vi "sv_Overall Level Plot (XY).vi"(6 "X axis selection":u16(ring)=2 items=["Time", "Revolution", "RPM"], 7 "reset? (True)":bool=TRUE, 8 "speed profile":T1 {"speed [RPM]" format="%.2f"; "time [s]" format="%.2f"}, 9 "samples/rev":dbl=1.0 format="%.2f", 11 "overall level (even angular)":dbl[][](array[numeric]) format="%.2f") -> (1 "X unit":string, 3 "overall level":cluster{"X":dbl[], "Y":dbl[]}[](array[cluster]) {"Y" format="%.2f"; "X" format="%.2f"})   [LabVIEW 2017, in "SoundVib_ContSweptSine.lvlib"]
uses:
  <vilib>/addons/Sound and Vibration/svt_Continuous Swept Sine/SoundVib_ContSweptSine.lvlib
  <vilib>/addons/Sound and Vibration/Order Analysis/Tach Process/SubVIs/speed profile.ctl
  <vilib>/Analysis/1siggen.llb/Ramp Pattern by Samples.vi
  <vilib>/Analysis/NI_AALBase.lvlib
  <vilib>/addons/Sound and Vibration/Order Analysis/Tach Process/SoundVib_TachProcess.lvlib
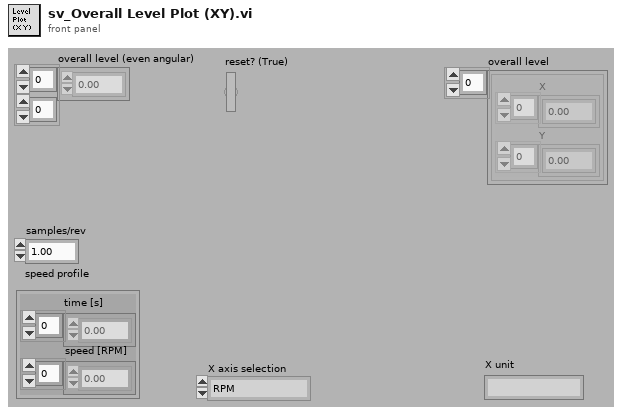
[diagram p1: front panel]
types:
  T1 = typedef "SoundVib_TachProcess.lvlib/speed profile.ctl" = cluster{"time [s]":dbl[], "speed [RPM]":dbl[]}
  T2 = cluster{"time [s]":dbl[], "overall level (even angular)":dbl[]}
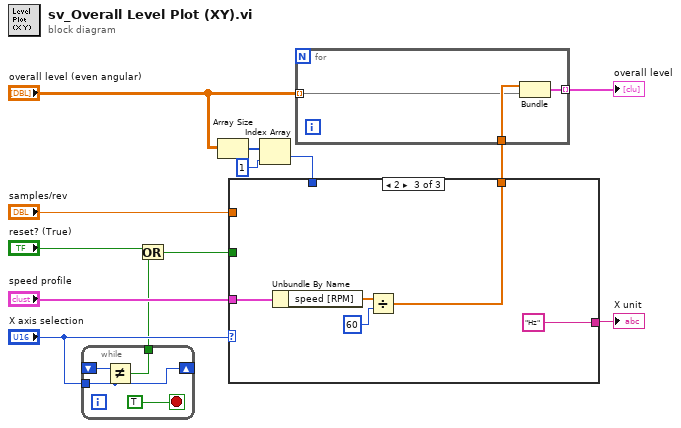
[diagram p0: block diagram]
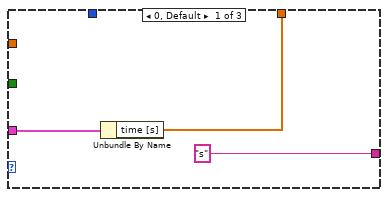
[diagram p2: hidden frame]
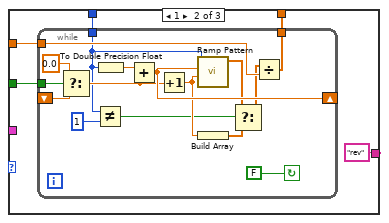
[diagram p3: hidden frame]
diagram:
  n1 = while {
    shift-right: [w15] -> _
    shift-left: _ -> [w16]
    tunnel: "X axis selection" -> [w15]
    tunnel: [w14] -> w1
    stop <- TRUE stop-if-true
    n2 = Not Equal?(x=w16, y=w15) -> (x != y?=w14:bool)
  }
  n3 = Or(x="reset? (True)", y=w1) -> (x .or. y?=w3:bool)
  n4 = Array Size(array="overall level (even angular)") -> (size(s)=w12:i32[])
  n5 = Index Array(array=w12, index=1) -> (element=w9:i32)
  n6 = case shown="2" "X axis selection" {
    tunnel: "speed profile" -> [w20 _ w46]
    tunnel: [w19 w25 w43] -> w10
    tunnel: w9 -> [_ w21 _]
    tunnel: "samples/rev" -> [_ w23 _]
    tunnel: ["s" "rev" "Hz"] -> w6
    tunnel: w3 -> [_ w22 _]
    frame 0, Default {
      n7 = Unbundle By Name(w20) -> ("time [s]"=w19:dbl[])
    }
    frame 1 {
      n8 = while {
        tunnel: [w41] -> w25
        tunnel: w23 -> [w40]
        tunnel: w22 -> [w38]
        shift-right: [w35] -> _
        shift-left: _ -> [w36]
        tunnel: w21 -> [w32]
        stop <- FALSE continue-if-true
        n9 = Select(t=0.0 ("f"), s=w38, f=w36) -> (s? t:f=w34:dbl)
        n10 = Not Equal?(x=w32, y=1) -> (x != y?=w30:bool)
        n11 = To Double Precision Float(number=w32) -> (double precision float=w26:dbl)
        n12 = Add(x=w26, y=w34) -> (x+y=w35:dbl)
        n13 = Increment(x=w34) -> (x+1=w31:dbl)
        n14 = call-poly <vilib>:"Ramp Pattern.vi"("start"=w31, "end"=w35, "samples"=w32) -> ("Ramp Pattern"=w29:dbl[])  [unwired: 7 in, 1 out]
        n15 = Build Array(w31) -> (w28:dbl[])
        n16 = Select(t=w29, s=w30, f=w28) -> (s? t:f=w27:dbl[])
        n17 = Divide(x=w27, y=w40) -> (x/y=w41:dbl[])
      }
    }
    frame 2 {
      n18 = Unbundle By Name(w46) -> ("speed [RPM]"=w45:dbl[])
      n19 = Divide(x=w45, y=60) -> (x/y=w43:dbl[])
    }
  }
  "X unit" <- w6
  n20 = for {
    tunnel: [w49] -> w7 mode=indexing
    tunnel: "overall level (even angular)" -> [w47] mode=indexing
    tunnel: w10 -> [w48]
    n21 = Bundle("time [s]"=w48, "overall level (even angular)"=w47) -> (w49:T2)  [unwired: 1 in]
  }
  "overall level" <- w7
